vi "Read_RootFolder Path.vi"(8 "error in (no error)":errorcluster, 11 "Process in":refnum<class "Process.lvclass">) -> (0 "error out":errorcluster, 2 "RootFolder Path":path, 3 "Process out":refnum<class "Process.lvclass">)   [LabVIEW 2013, in "Process.lvclass"]
uses:
  Process.lvclass
  Process.lvclass/Process.ctl
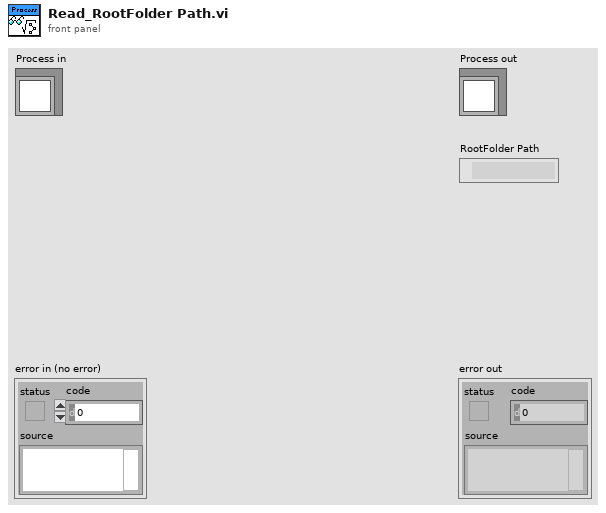
[diagram p1: front panel]
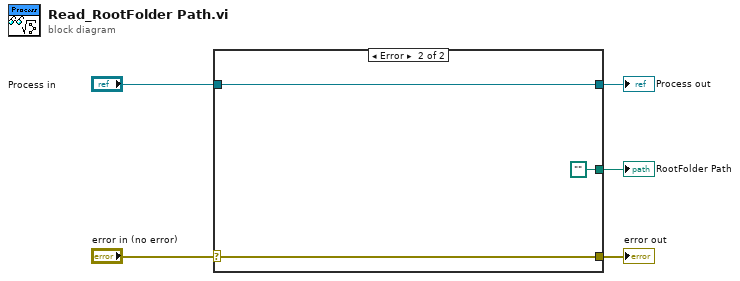
[diagram p0: block diagram]
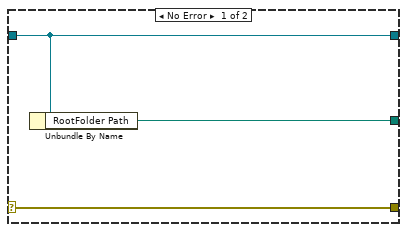
[diagram p2: hidden frame]
diagram:
  n1 = case shown="Error" "error in (no error)" {
    selector: "error in (no error)" -> [w8 w10]
    tunnel: [w8 w10] -> w4
    tunnel: [w7 w11] -> w2
    tunnel: "Process in" -> [w7 w11]
    tunnel: [w6 path ""] -> w1
    frame No Error {
      n2 = Unbundle By Name(w7) -> ("RootFolder Path"=w6:path)
    }
    frame Error {
    }
  }
  "error out" <- w4
  "Process out" <- w2
  "RootFolder Path" <- w1
